vi "Publish Driver Selftest.vi"(8 "error in (no error)":errorcluster, 11 "CS++DeviceActor in":refnum<class "CS++DeviceActor.lvclass">) -> (0 "error out":errorcluster, 3 "CS++DeviceActor out":refnum<class "CS++DeviceActor.lvclass">)   [LabVIEW 2013, in "CS++DeviceActor.lvlib" / "CS++DeviceActor.lvclass"]
doc: "Publish driver selftest results."
uses:
  CS++DeviceActor.lvclass
  Classes/CS++ProcessVariables/ProcessVariable/PV.lvclass
  CS++DeviceActor.lvclass/CS++DeviceActor.ctl
  Classes/CS++ProcessVariables/PVConnection/PVConnection.lvclass
  Classes/CS++ProcessVariables/ProcessVariable/PV.lvclass/PV.ctl
  Classes/CS++ProcessVariables/ProcessVariable/Write Data.vi
  Classes/CS++ProcessVariables/ProcessVariable/Write Timestamp.vi
  Classes/CS++ProcessVariables/ProcessVariable/Write Quality.vi
  Classes/CS++ProcessVariables/ProcessVariable/Write status.vi
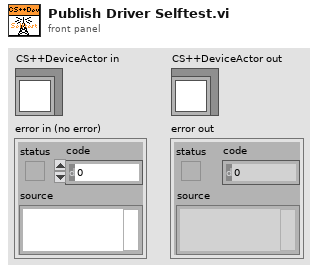
[diagram p1: front panel]
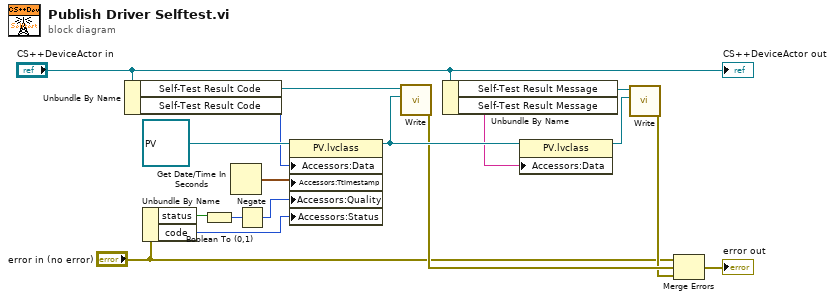
[diagram p0: block diagram]
diagram:
  n1 = Unbundle By Name("CS++DeviceActor in") -> ("Self-Test Result Code"=w17:refnum<class "PVConnection.lvclass">, "Self-Test Result Code"=w15:i32)
  n2 = Unbundle By Name("error in (no error)") -> ("status"=w13:bool, "code"=w10:i32)
  n3 = Boolean To (0,1)(Boolean=w13) -> (0, 1=w12:i16)
  n4 = Get Date/Time In Seconds() -> (seconds since 1Jan1904=w14:timestamp)
  n5 = Negate(x=w12) -> (-x=w11:i16)
  n6 = property class="PV.lvclass"(reference=refnum<class "PV.lvclass"> refnum ("CS++ProcessVariables.lvlib:PV.lvclass"), "Accessors:Data"=w15, "Accessors:Ttimestamp"=w14, "Accessors:Quality"=w11, "Accessors:Status"=w10) -> (reference out=w8:refnum<class "PV.lvclass">)  [unwired: 1 in, 1 out]
  n7 = call-dynamic "Write.vi"("PV"=w8, "PVConnection in"=w17) -> ("error out"=w5:errorcluster)  [unwired: 8 in, 1 out]
  n8 = Unbundle By Name("CS++DeviceActor in") -> ("Self-Test Result Message"=w9:refnum<class "PVConnection.lvclass">, "Self-Test Result Message"=w7:string)
  n9 = property class="PV.lvclass"(reference=w8, "Accessors:Data"=w7) -> (reference out=w1:refnum<class "PV.lvclass">)  [unwired: 1 in, 1 out]
  n10 = call-dynamic "Write.vi"("PV"=w1, "PVConnection in"=w9) -> ("error out"=w4:errorcluster)  [unwired: 8 in, 1 out]
  n11 = Merge Errors("error in (no error)", w5, w4) -> (→"error out":errorcluster)
  "CS++DeviceActor out" <- "CS++DeviceActor in"
